vi "PL_Spectrum.vi"() -> ()   [LabVIEW 2012]
uses:
  <vilib>/Utility/file.llb/Write To Spreadsheet File (DBL).vi
  <vilib>/Instr/_visa.llb/VISA Configure Serial Port (Instr).vi
  <vilib>/Analysis/baseanly.llb/Mean (DBL).vi
  <vilib>/Analysis/NI_AALBase.lvlib
panel:
  out "XY Graph":cluster{"Y":dbl[], "Y":dbl[]}[](graph)
  in  "End Wavelength (nm)":dbl
  in  "Start Wavelength (nm)":dbl
  in  "Resolution (nm)":dbl
  in  "Detector Input":T1
  in  "stop (T)":bool=TRUE
  in  "Resource name":refnum<visa-resource-name>
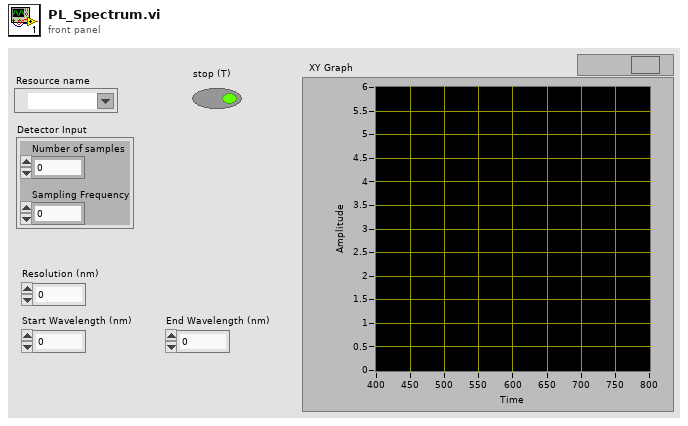
[diagram p1: front panel]
types:
  T1 = cluster{"Number of samples":i32, "Sampling Frequency":dbl}
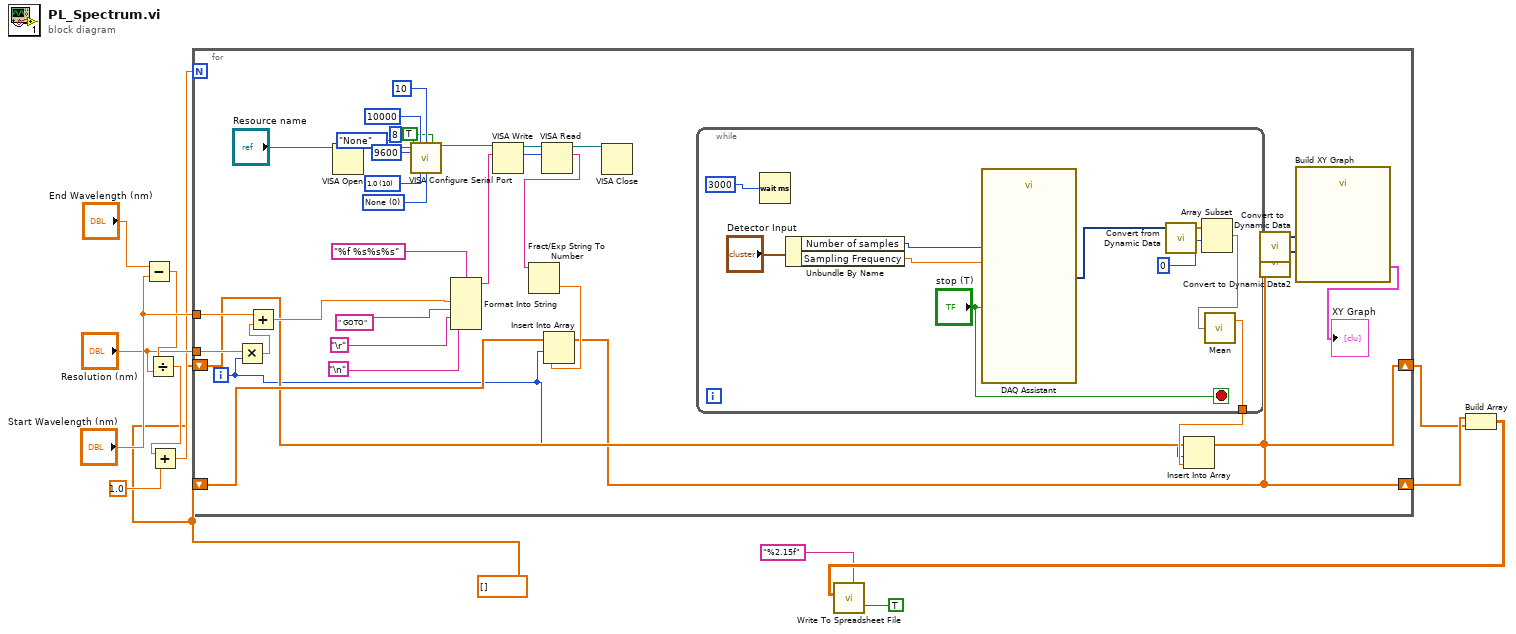
[diagram p0: block diagram]
diagram:
  w5 = dbl[] [] ("array")
  n1 = Subtract(x="End Wavelength (nm)", y="Start Wavelength (nm)") -> (x-y=w10:dbl)
  n2 = Divide(x=w10, y="Resolution (nm)") -> (x/y=w8:dbl)
  n3 = Add(x=w8, y=1.0) -> (x+y=w6:dbl)
  n4 = for {
    N: w6 -> [_]
    shift-right: [w17] -> w4
    shift-left: w5 -> [w25]
    tunnel: "Resolution (nm)" -> [w24]
    tunnel: "Start Wavelength (nm)" -> [w23]
    shift-right: [w15] -> w3
    shift-left: w5 -> [w20]
    i -> [w19]
    w36 = u16 0 items=["None", "XON/XOFF", "RTS/CTS", "XON/XOFF & RTS/CTS", "DTR/DSR", "XON/XOFF & DTR/DSR"] ("flow control (0:none)")
    w37 = u16 10 items=["1.0"=10, "1.5"=15, "2.0"=20] ("stop bits (10: 1 bit)")
    n5 = Multiply(x=w24, y=w19) -> (x*y=w26:dbl)
    n6 = Add(x=w23, y=w26) -> (x+y=w27:dbl)
    n7 = VISA Open(VISA resource name="Resource name") -> (VISA resource name=w41:refnum<visa-resource-name>)  [unwired: 4 in, 1 out]
    n8 = call-poly "VISA Configure Serial Port"("VISA resource name"=w41, "timeout (10sec)"=u32 10000, "termination char\n(0xA = '\\n' = LF)"=u8 10 ("termination char\n(0xA = '\\n' = LF)"), "Enable Termination\nChar (T)"=TRUE ("Enable Termination\nChar (T)"), "baud rate (9600)"=u32 9600, "data bits (8)"=u16 8, "parity (0:none)"=enum16{"None", "Odd", "Even", "Mark", "Space"}."None", "stop bits (10: 1 bit)"=w37, "flow control (0:none)"=w36) -> ("VISA resource name out"=w31:refnum<visa-resource-name>)  [unwired: 5 in, 1 out]
    n9 = Format Into String(format string="%f %s%s%s", w27, " GOTO" ("String"), "\r", "\n") -> (resulting string=w32:string)  [unwired: 2 in, 1 out]
    n10 = VISA Write(VISA resource name=w31, write buffer=w32) -> (VISA resource name out=w43:refnum<visa-resource-name>, return count=w42:u32)  [unwired: 1 in, 1 out]
    n11 = VISA Read(VISA resource name=w43, byte count=w42) -> (VISA resource name out=w29:refnum<visa-resource-name>, read buffer=w30:string)  [unwired: 1 in, 2 out]
    n12 = Fract/Exp String To Number(string=w30) -> (number=w22:dbl)  [unwired: 3 in, 1 out]
    n13 = Insert Into Array(array=w25, index=w19, new element=w22) -> (w17:dbl[])
    n14 = VISA Close(VISA resource name=w29) -> ()  [unwired: 1 in, 1 out]
    n15 = while {
      tunnel: [w53] -> w21
      stop <- "stop (T)" stop-if-true
      n16 = Wait (ms)(milliseconds to wait=u32 3000) -> ()  [unwired: 1 out]
      n17 = Unbundle By Name("Detector Input") -> ("Number of samples"=w50:i32, "Sampling Frequency"=w49:dbl)
      n18 = call "DAQ Assistant"("rate"=w49, "number of samples"=w50, "stop (T)"="stop (T)") -> ("data"=w57:dynamicdata)  [unwired: 14 in, 2 out]
      n19 = call "Convert from Dynamic Data"("Dynamic Data Type"=w57) -> ("Array"=w56:dbl[])  [unwired: 3 in]
      n20 = Array Subset(array=w56, index=0) -> (w55:dbl[])  [unwired: 1 in]
      n21 = call-poly <vilib>:"Mean.vi"("X"=w55) -> ("mean"=w53:dbl)  [unwired: 1 out]
    }
    n22 = Insert Into Array(array=w20, index=w19, new element=w21) -> (w15:dbl[])
    n23 = call "Convert to Dynamic Data"("Array"=w17) -> ("Dynamic Data Type"=w16:dynamicdata)  [unwired: 3 in]
    n24 = call "Convert to Dynamic Data2"("Array"=w15) -> ("Dynamic Data Type"=w14:dynamicdata)  [unwired: 3 in]
    n25 = call "Build XY Graph"("Y Input"=w14, "X Input"=w16) -> ("XY Graph"=→"XY Graph":cluster{"Y":dbl[], "Y":dbl[]}[])  [unwired: 8 in, 1 out]
  }
  n26 = Build Array(w4, w3) -> (w2:dbl[][])
  n27 = call-poly <vilib>:"Write To Spreadsheet File.vi"("transpose? (no:F)"=TRUE, "format (%.3f)"="%2.15f" ("format string"), "2D data"=w2) -> ()  [unwired: 5 in, 1 out]
